vi "write_mcsmode_command.vi"(10 "sequential mode":bool, 11 "dual mcs":bool) -> (3 "String":string)   [LabVIEW 2015]
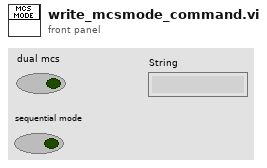
[diagram p1: front panel]
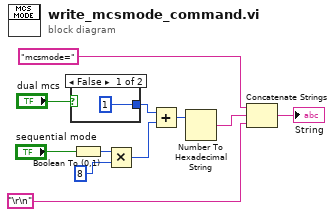
[diagram p0: block diagram]
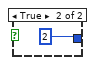
[diagram p2: hidden frame]
diagram:
  n1 = case shown="False" "dual mcs" {
    tunnel: [1 2] -> w5
    frame False {
    }
    frame True {
    }
  }
  n2 = Boolean To (0,1)(Boolean="sequential mode") -> (0, 1=w8:i16)
  n3 = Multiply(x=w8, y=i16 8) -> (x*y=w4:i16)
  n4 = Add(x=w5, y=w4) -> (x+y=w3:i32)
  n5 = Number To Hexadecimal String(2:w3) -> (0:w2:string)  [unwired: 1 in]
  n6 = Concatenate Strings("mcsmode=", w2, "\r\n") -> (→"String":string)
